vi "compare_and_convert_fxp_32_16_to_i32.vi"(2 "low":fxp<+/-,32,16>, 3 "fxp32_16":fxp<+/-,32,16>, 4 "high":fxp<+/-,32,16>) -> (0 "out_of_range":bool, 1 "32bit integer":i32)   [LabVIEW 2018]
uses:
  <vilib>/rvi/FXPMathLib/FxpInterpret/XNode/nifxpmath_Interpret.xnode
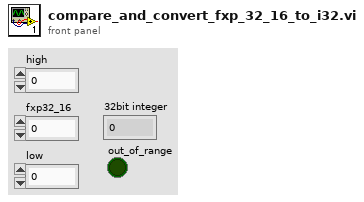
[diagram p1: front panel]
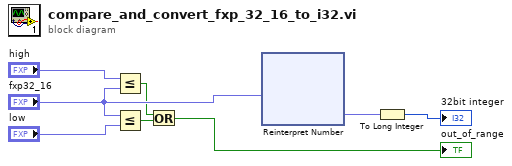
[diagram p0: block diagram]
diagram:
  n1 = Less Or Equal?(x="high", y="fxp32_16") -> (x <= y?=w2:bool)
  n2 = Less Or Equal?(x="fxp32_16", y="low") -> (x <= y?=w3:bool)
  n3 = Or(x=w2, y=w3) -> (x .or. y?=→"out_of_range":bool)
  n4 = xnode "Reinterpret Number"("x"="fxp32_16") -> ("y"=w8:fxp<+/-,32,32>)
  n5 = To Long Integer(number=w8) -> (32bit integer=→"32bit integer":i32)
